vi "Tool STroker analog Variables.vi"(11 "error in (no error)":errorcluster, 12 "Tool folder name":string) -> (15 "error out":errorcluster)   [LabVIEW 2011]
uses:
  Measurments Handling/Fixed Digital Channel Definition.ctl
  Measurments Handling/Update frequensies.ctl
  Measurments Handling/Channel catagory Enum.ctl
  Variable List Stroker Digital2.ctl
  Tool/Extended channel identifier for tool.ctl
  Variable List Stroker Analog2.ctl
  Measurments Handling/Fixed Analog Channel Definition.ctl
  Measurments Handling/Units/Quantity enum.ctl
  Measurments Handling/Scaling.ctl
  <vilib>/Utility/VariantDataType/GetNumericInfo.vi
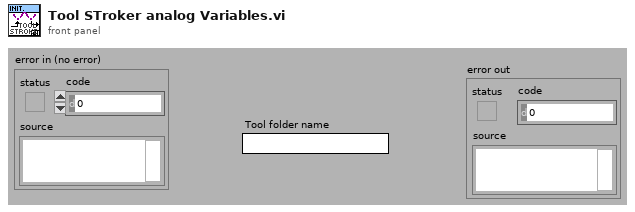
[diagram p1: front panel]
types:
  T1 = typedef "Variable List Stroker Analog2.ctl" = enum16{"Tool max Temperature", "Tool (Solenoid) Temperature", "Tool supply Voltage", "Tool (Controller) Current", "Tool Acceleration X", "Tool Acceleration Y", "Tool Acceleration Z", "Tool (Controller) Temperature", "Tool Acceleration Sum", "Tool Inclination", "Tool Rotation", "Tool Stroke Extension", "Tool GP Sensor 1", "Tool GP Sensor 2", "Tool (Pressure 1) Temperature", "Tool Pressure 1", "Tool (Pressure 2) Temperature", "Tool Pressure 2", "Do not use (SIF)", "Do not use (SOF)", "Stroke Force"}
  T2 = typedef "Fixed Analog Channel Definition.ctl" = cluster{"ID":u16, "Name":string, "Quantity":T3, "Unit":string, "Maximum upd":T4, "Comment":string, "Help file Name":string, "Help file Section ":string, "Category":T5, "User adjustable Scaling":bool, "Default Scaling":T6, "In use":bool, "Default Unit":i32}
  T3 = typedef "Quantity enum.ctl" = enum16{"Acceleration", "Angle", "Current", "Force", "Distance", "Pressure", "Resistance", "Rotational Speed", "Speed", "Temperature", "Tension", "Torque", "Voltage", "Weight"}
  T4 = typedef "Update frequensies.ctl" = enum16{"2 Hz", "1 Hz", "0.1 Hz"}
  T5 = typedef "Channel catagory Enum.ctl" = enum16{"No Category", "Power", "Temperature", "Pressure"}
  T6 = typedef "Scaling.ctl" = cluster{"Gain":dbl, "Offset":dbl}
  T7 = typedef "Extended channel identifier for tool.ctl" = cluster{"ID":T1, "Variable Defenition":T2}
  T8 = typedef "Fixed Digital Channel Definition.ctl" = cluster{"ID":u16, "Name":string, "NA Text":string, "Off Text":string, "On Text":string, "Maximum upd":T4, "Comment":string, "Help file Name":string, "Help file Section ":string, "Catagory":T5, "In use":bool}
  T9 = typedef "Variable List Stroker Digital2.ctl" = enum16{"Tool Stroke enable Valve", "Tool Stroke direction Valve", "Tool Anchor Valve", "Tool Relay 1", "Tool Relay 2", "Tool node pressure 1", "Tool node pressure 2", "Tool node solenoid", "Tool High G Monitoring", "Tool High G Recording", "Tool High G Data ready", "Tool Anchor(Not Available)", "Tool error Controller", "Tool error Pressure 1", "Tool error Pressure 2", "Tool error Solenoid", "Tool stopped Controller", "Tool stopped Pressure 1", "Tool stopped Pressure 2", "Tool stopped Solenoid", "Stroke Target seeking", "Stroke Moving Out", "Stroke Moving Inn", "Stroke valves set for Out", "Stroke valves set for In", "Stroke In (force)", "Stroke Out (force)", "Stroke Force decreasing(in)", "Stroke Force decreasing(out)", "Stroke Force change not correct", "Stroke SLIPS established P1", "Stroke SLIPS established P2", "Stroke SLIPS established"}
  T10 = typedef "User Setting DigitalChannel.ctl" = cluster{"Responses":cluster{"Technical Error (NA)":T11, "OFF / FALSE":T13, "ON / TRUE":T13}}
  T11 = typedef "Alarm Responce.ctl" = cluster{"Action":T12, "Alarm":bool}
  T12 = typedef "Action List.ctl" = u16
  T13 = typedef "Alarm Responce dig.ctl" = cluster{"Action":T12, "Alarm":bool, "Exclamation":bool}
  T14 = typedef "User Setting Analog Channel Bg.ctl" = cluster{"Scaling":T6, "Limits and responces":T15, "Allow Graph selection by user":bool, "Unit":u16}
  T15 = typedef "Alarm Setup Analog.ctl" = cluster{"Technical Error(NA)":T11, "LL":T11, "L":T11, "H":T11, "HH":T11, "Limits":T16}
  T16 = typedef "Limits.ctl" = cluster{"LL":dbl, "L":dbl, "H":dbl, "HH":dbl}
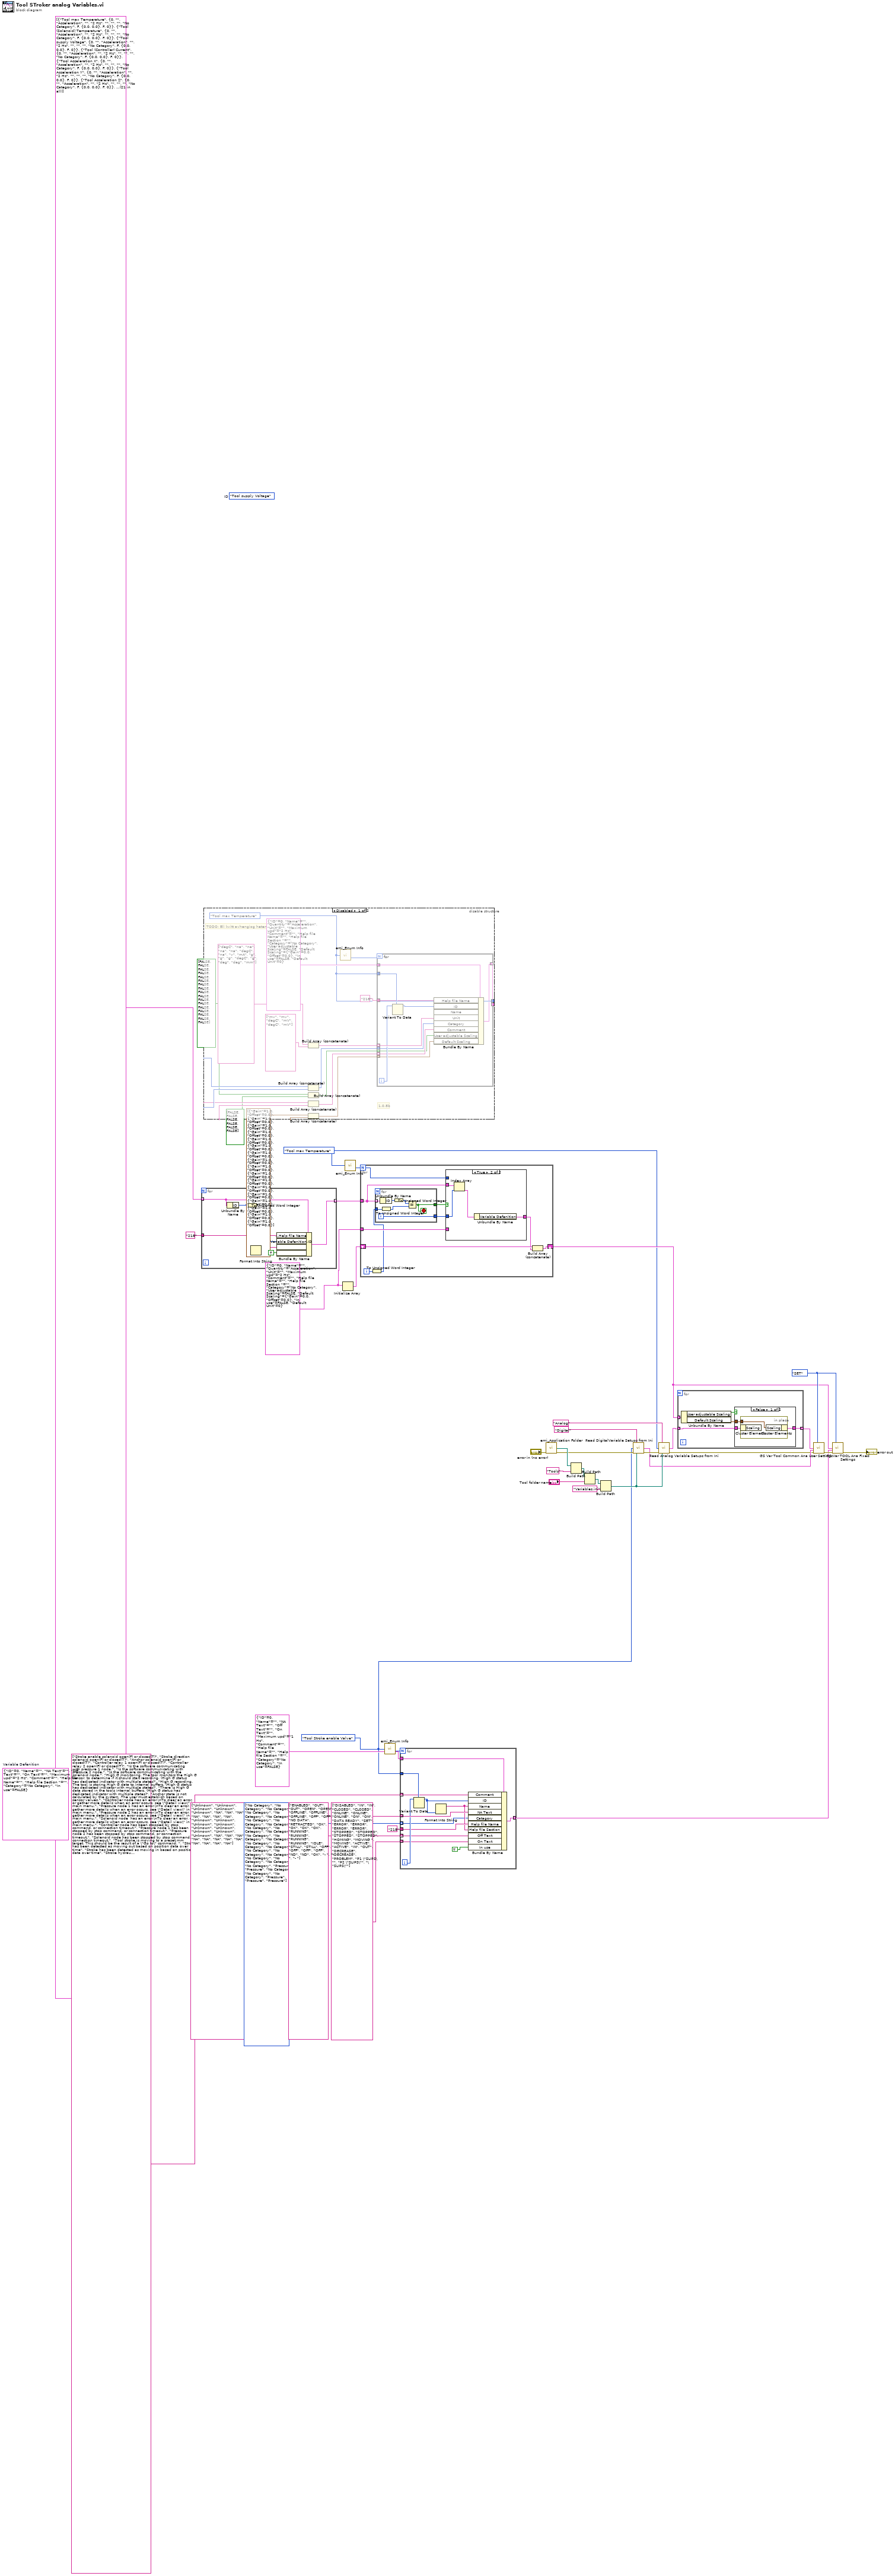
[diagram p0: block diagram]
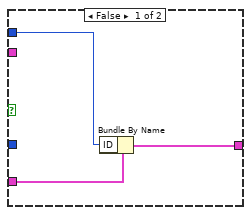
[diagram p2: hidden frame]
diagram:
  (unwired) Variable_List_Stroker_Analog2."Tool supply Voltage"  # ID
  w3 = T2 {"ID"=0, "Name"="", "Quantity"=enum."Acceleration", "Unit"="", "Maximum upd"=enum."2 Hz", "Comment"="", "Help file Name"="", "Help file Section "="", "Category"=enum."No Category", "User adjustable Scaling"=FALSE, "Default Scaling"={"Gain"=0.0, "Offset"=0.0}, "In use"=FALSE, "Default Unit"=0} ("Variable Defenition")
  w1 = Variable_List_Stroker_Analog2."Tool max Temperature" ("Action")
  (unwired) T8 {"ID"=0, "Name"="", "NA Text"="", "Off Text"="", "On Text"="", "Maximum upd"=enum."2 Hz", "Comment"="", "Help file Name"="", "Help file Section "="", "Catagory"=enum."No Category", "In use"=FALSE}  # Variable Defenition
  w22 = T5[] [enum."No Category", enum."No Category", enum."No Category", enum."No Category", enum."No Category", enum."No Category", enum."No Category", enum."No Category", enum."No Category", enum."No Category", enum."No Category", enum."No Category", enum."No Category", enum."No Category", enum."No Category", enum."No Category", enum."No Category", enum."No Category", enum."No Category", enum."No Category", enum."No Category", enum."No Category", enum."No Category", enum."No Category", enum."No Category", enum."Pressure", enum."Pressure", enum."No Category", enum."No Category", enum."No Category", enum."Pressure", enum."Pressure", enum."Pressure"] items=["No Category", "Power", "Temperature", "Pressure"]
  w14 = Variable_List_Stroker_Digital2."Tool Stroke enable Valve" ("Action")
  w29 = enum16{"GET", "SET"}."SET" ("Action(GET)")
  n1 = for {
    tunnel: T7[] [{"ID"=enum."Tool max Temperature", "Variable Defenition"={"ID"=0, "Name"="", "Quantity"=enum."Acceleration", "Unit"="", "Maximum upd"=enum."2 Hz", "Comment"="", "Help file Name"="", "Help file Section "="", "Category"=enum."No Category", "User adjustable Scaling"=FALSE, "Default Scaling"={"Gain"=0.0, "Offset"=0.0}, "In use"=FALSE, "Default Unit"=0}}, {"ID"=enum."Tool (Solenoid) Temperature", "Variable Defenition"={"ID"=0, "Name"="", "Quantity"=enum."Acceleration", "Unit"="", "Maximum upd"=enum."2 Hz", "Comment"="", "Help file Name"="", "Help file Section "="", "Category"=enum."No Category", "User adjustable Scaling"=FALSE, "Default Scaling"={"Gain"=0.0, "Offset"=0.0}, "In use"=FALSE, "Default Unit"=0}}, {"ID"=enum."Tool supply Voltage", "Variable Defenition"={"ID"=0, "Name"="", "Quantity"=enum."Acceleration", "Unit"="", "Maximum upd"=enum."2 Hz", "Comment"="", "Help file Name"="", "Help file Section "="", "Category"=enum."No Category", "User adjustable Scaling"=FALSE, "Default Scaling"={"Gain"=0.0, "Offset"=0.0}, "In use"=FALSE, "Default Unit"=0}}, {"ID"=enum."Tool (Controller) Current", "Variable Defenition"={"ID"=0, "Name"="", "Quantity"=enum."Acceleration", "Unit"="", "Maximum upd"=enum."2 Hz", "Comment"="", "Help file Name"="", "Help file Section "="", "Category"=enum."No Category", "User adjustable Scaling"=FALSE, "Default Scaling"={"Gain"=0.0, "Offset"=0.0}, "In use"=FALSE, "Default Unit"=0}}, {"ID"=enum."Tool Acceleration X", "Variable Defenition"={"ID"=0, "Name"="", "Quantity"=enum."Acceleration", "Unit"="", "Maximum upd"=enum."2 Hz", "Comment"="", "Help file Name"="", "Help file Section "="", "Category"=enum."No Category", "User adjustable Scaling"=FALSE, "Default Scaling"={"Gain"=0.0, "Offset"=0.0}, "In use"=FALSE, "Default Unit"=0}}, {"ID"=enum."Tool Acceleration Y", "Variable Defenition"={"ID"=0, "Name"="", "Quantity"=enum."Acceleration", "Unit"="", "Maximum upd"=enum."2 Hz", "Comment"="", "Help file Name"="", "Help file Section "="", "Category"=enum."No Category", "User adjustable Scaling"=FALSE, "Default Scaling"={"Gain"=0.0, "Offset"=0.0}, "In use"=FALSE, "Default Unit"=0}}, {"ID"=enum."Tool Acceleration Z", "Variable Defenition"={"ID"=0, "Name"="", "Quantity"=enum."Acceleration", "Unit"="", "Maximum upd"=enum."2 Hz", "Comment"="", "Help file Name"="", "Help file Section "="", "Category"=enum."No Category", "User adjustable Scaling"=FALSE, "Default Scaling"={"Gain"=0.0, "Offset"=0.0}, "In use"=FALSE, "Default Unit"=0}}, {"ID"=enum."Tool (Controller) Temperature", "Variable Defenition"={"ID"=0, "Name"="", "Quantity"=enum."Acceleration", "Unit"="", "Maximum upd"=enum."2 Hz", "Comment"="", "Help file Name"="", "Help file Section "="", "Category"=enum."No Category", "User adjustable Scaling"=FALSE, "Default Scaling"={"Gain"=0.0, "Offset"=0.0}, "In use"=FALSE, "Default Unit"=0}}, {"ID"=enum."Tool Acceleration Sum", "Variable Defenition"={"ID"=0, "Name"="", "Quantity"=enum."Acceleration", "Unit"="", "Maximum upd"=enum."2 Hz", "Comment"="", "Help file Name"="", "Help file Section "="", "Category"=enum."No Category", "User adjustable Scaling"=FALSE, "Default Scaling"={"Gain"=0.0, "Offset"=0.0}, "In use"=FALSE, "Default Unit"=0}}, {"ID"=enum."Tool Inclination", "Variable Defenition"={"ID"=0, "Name"="", "Quantity"=enum."Acceleration", "Unit"="", "Maximum upd"=enum."2 Hz", "Comment"="", "Help file Name"="", "Help file Section "="", "Category"=enum."No Category", "User adjustable Scaling"=FALSE, "Default Scaling"={"Gain"=0.0, "Offset"=0.0}, "In use"=FALSE, "Default Unit"=0}}, {"ID"=enum."Tool Rotation", "Variable Defenition"={"ID"=0, "Name"="", "Quantity"=enum."Acceleration", "Unit"="", "Maximum upd"=enum."2 Hz", "Comment"="", "Help file Name"="", "Help file Section "="", "Category"=enum."No Category", "User adjustable Scaling"=FALSE, "Default Scaling"={"Gain"=0.0, "Offset"=0.0}, "In use"=FALSE, "Default Unit"=0}}, {"ID"=enum."Tool Stroke Extension", "Variable Defenition"={"ID"=0, "Name"="", "Quantity"=enum."Acceleration", "Unit"="", "Maximum upd"=enum."2 Hz", "Comment"="", "Help file Name"="", "Help file Section "="", "Category"=enum."No Category", "User adjustable Scaling"=FALSE, "Default Scaling"={"Gain"=0.0, "Offset"=0.0}, "In use"=FALSE, "Default Unit"=0}}, {"ID"=enum."Tool GP Sensor 1", "Variable Defenition"={"ID"=0, "Name"="", "Quantity"=enum."Acceleration", "Unit"="", "Maximum upd"=enum."2 Hz", "Comment"="", "Help file Name"="", "Help file Section "="", "Category"=enum."No Category", "User adjustable Scaling"=FALSE, "Default Scaling"={"Gain"=0.0, "Offset"=0.0}, "In use"=FALSE, "Default Unit"=0}}, {"ID"=enum."Tool GP Sensor 2", "Variable Defenition"={"ID"=0, "Name"="", "Quantity"=enum."Acceleration", "Unit"="", "Maximum upd"=enum."2 Hz", "Comment"="", "Help file Name"="", "Help file Section "="", "Category"=enum."No Category", "User adjustable Scaling"=FALSE, "Default Scaling"={"Gain"=0.0, "Offset"=0.0}, "In use"=FALSE, "Default Unit"=0}}, {"ID"=enum."Tool (Pressure 1) Temperature", "Variable Defenition"={"ID"=0, "Name"="", "Quantity"=enum."Acceleration", "Unit"="", "Maximum upd"=enum."2 Hz", "Comment"="", "Help file Name"="", "Help file Section "="", "Category"=enum."No Category", "User adjustable Scaling"=FALSE, "Default Scaling"={"Gain"=0.0, "Offset"=0.0}, "In use"=FALSE, "Default Unit"=0}}, {"ID"=enum."Tool Pressure 1", "Variable Defenition"={"ID"=0, "Name"="", "Quantity"=enum."Acceleration", "Unit"="", "Maximum upd"=enum."2 Hz", "Comment"="", "Help file Name"="", "Help file Section "="", "Category"=enum."No Category", "User adjustable Scaling"=FALSE, "Default Scaling"={"Gain"=0.0, "Offset"=0.0}, "In use"=FALSE, "Default Unit"=0}}, {"ID"=enum."Tool (Pressure 2) Temperature", "Variable Defenition"={"ID"=0, "Name"="", "Quantity"=enum."Acceleration", "Unit"="", "Maximum upd"=enum."2 Hz", "Comment"="", "Help file Name"="", "Help file Section "="", "Category"=enum."No Category", "User adjustable Scaling"=FALSE, "Default Scaling"={"Gain"=0.0, "Offset"=0.0}, "In use"=FALSE, "Default Unit"=0}}, {"ID"=enum."Tool Pressure 2", "Variable Defenition"={"ID"=0, "Name"="", "Quantity"=enum."Acceleration", "Unit"="", "Maximum upd"=enum."2 Hz", "Comment"="", "Help file Name"="", "Help file Section "="", "Category"=enum."No Category", "User adjustable Scaling"=FALSE, "Default Scaling"={"Gain"=0.0, "Offset"=0.0}, "In use"=FALSE, "Default Unit"=0}}, {"ID"=enum."Do not use (SIF)", "Variable Defenition"={"ID"=0, "Name"="", "Quantity"=enum."Acceleration", "Unit"="", "Maximum upd"=enum."2 Hz", "Comment"="", "Help file Name"="", "Help file Section "="", "Category"=enum."No Category", "User adjustable Scaling"=FALSE, "Default Scaling"={"Gain"=0.0, "Offset"=0.0}, "In use"=FALSE, "Default Unit"=0}}, {"ID"=enum."Do not use (SOF)", "Variable Defenition"={"ID"=0, "Name"="", "Quantity"=enum."Acceleration", "Unit"="", "Maximum upd"=enum."2 Hz", "Comment"="", "Help file Name"="", "Help file Section "="", "Category"=enum."No Category", "User adjustable Scaling"=FALSE, "Default Scaling"={"Gain"=0.0, "Offset"=0.0}, "In use"=FALSE, "Default Unit"=0}}, {"ID"=enum."Stroke Force", "Variable Defenition"={"ID"=0, "Name"="", "Quantity"=enum."Acceleration", "Unit"="", "Maximum upd"=enum."2 Hz", "Comment"="", "Help file Name"="", "Help file Section "="", "Category"=enum."No Category", "User adjustable Scaling"=FALSE, "Default Scaling"={"Gain"=0.0, "Offset"=0.0}, "In use"=FALSE, "Default Unit"=0}}] -> [w43] mode=indexing
    tunnel: "218" ("Help file Name") -> [w44]
    tunnel: [w38] -> w5 mode=indexing
    n2 = Unbundle By Name(w43) -> ("ID"=w41:T1)
    n3 = To Unsigned Word Integer(number=w41) -> (unsigned 16bit integer=w42:u16)
    n4 = Format Into String(w41) -> (resulting string=w40:string)  [unwired: 3 in, 1 out]
    n5 = Bundle By Name(cluster=w43, "Variable Defenition.Help file Name"=w44, "Variable Defenition.ID"=w42, "Variable Defenition.Name"=w40, "Variable Defenition.In use"=TRUE) -> (w38:T7)
  }
  n6 = disable-structure shown="Disabled" {
    disable-tunnel: [w46 _] -> _
    disable-tunnel: [w45 _] -> _
    frame Disabled {
      w58 = T5[] [enum."No Category", enum."No Category", enum."Temperature", enum."Pressure", enum."Temperature", enum."Pressure"] items=["No Category", "Power", "Temperature", "Pressure"]
      w59 = T5[] [enum."Temperature", enum."No Category", enum."No Category", enum."No Category", enum."No Category", enum."Temperature", enum."No Category", enum."Power", enum."Power", enum."No Category", enum."No Category", enum."No Category", enum."Temperature", enum."No Category", enum."No Category", enum."No Category", enum."No Category"] items=["No Category", "Power", "Temperature", "Pressure"]
      w45 = Variable_List_Stroker_Analog2."Tool max Temperature" ("Action")
      # "1.0.8b"
      # "TODO: Bli kvitt avhengiog heten av denne"
      n7 = Build Array (concatenate)(string[] ["degC", "na", "na", "na", "na", "degC", "na", "v", "mA", "g", "g", "g", "degC", "g", "deg", "deg", "mm"], string[] ["mv", "mv", "degC", "mV", "degC", "mV"]) -> (w61:string[])
      n8 = Build Array (concatenate)(w59, w58) -> (w54:T5[])
      n9 = Build Array (concatenate)(bool[] [FALSE, FALSE, FALSE, FALSE, FALSE, FALSE, FALSE, FALSE, FALSE, FALSE, FALSE, FALSE, FALSE, FALSE, FALSE, FALSE, FALSE], bool[] [FALSE, FALSE, FALSE, FALSE, FALSE, FALSE]) -> (w51:bool[])
      n10 = Build Array (concatenate)(string[] ["The Highest temperature currently beeing measured in the tool.\nIf data from any of the tools temperature sensors is not reporting data, this is reported as Not Available.", "Not available\n", "Not available\n", "Not available\n", "Not available\n", "Temperature of the Solonoid electronics", "Not availabe\nThe Downhole Power Supply Temperature", "The Downhole tool's Controller board input voltage", "The Downhole tool's controller board input current", "The Downhole tool's controller board Acceleromter X axis. Used to determin heading", "The Downhole tool's controller board Acceleromter Y axis. Used to determin heading", "The Downhole tool's controller board Acceleromter Z axis. Used to determin heading", "The Downhole tool's controller board temperature", "Sum of the accelerations detected by the Downhole tool processor board", "Tool inclination as calculated by the controller board's accelerometer", "Tool rotation as calculated by the controller board's accelerometer", "Not available\nTool rotational speed  as calculated by the controller board's accelerometer"], string[] ["Tool Controller AI 24bit bridge sensor 1", "Tool Controller AI 24bit bridge sensor 2", "Pressure node 1 temperature", "Pressure node 1, pressure (shown in mV input of the sensor)", "Pressure node 2 temperature", "Pressure node 2, pressure (shown in mV input of the sensor)"]) -> (w55:string[])
      n11 = Build Array (concatenate)(T6[] [{"Gain"=1.0, "Offset"=0.0}, {"Gain"=1.0, "Offset"=0.0}, {"Gain"=1.0, "Offset"=0.0}, {"Gain"=1.0, "Offset"=0.0}, {"Gain"=1.0, "Offset"=0.0}, {"Gain"=1.0, "Offset"=0.0}, {"Gain"=1.0, "Offset"=0.0}, {"Gain"=1.0, "Offset"=0.0}, {"Gain"=1.0, "Offset"=0.0}, {"Gain"=1.0, "Offset"=0.0}, {"Gain"=1.0, "Offset"=0.0}, {"Gain"=1.0, "Offset"=0.0}, {"Gain"=1.0, "Offset"=0.0}, {"Gain"=1.0, "Offset"=0.0}, {"Gain"=1.0, "Offset"=0.0}, {"Gain"=1.0, "Offset"=0.0}, {"Gain"=1.0, "Offset"=0.0}], T6[] [{"Gain"=1.0, "Offset"=0.0}, {"Gain"=1.0, "Offset"=0.0}, {"Gain"=1.0, "Offset"=0.0}, {"Gain"=1.0, "Offset"=0.0}, {"Gain"=1.0, "Offset"=0.0}, {"Gain"=1.0, "Offset"=0.0}]) -> (w48:T6[])
      n12 = call "emi_Enum Info.vi"("Enum"=w45) -> ("Numb Elements"=w62:i32)  [unwired: 11 in, 3 out]
      n13 = for {
        N: w62 -> [_]
        tunnel: w45 -> [w76]
        tunnel: T2 {"ID"=0, "Name"="", "Quantity"=enum."Acceleration", "Unit"="", "Maximum upd"=enum."2 Hz", "Comment"="", "Help file Name"="", "Help file Section "="", "Category"=enum."No Category", "User adjustable Scaling"=FALSE, "Default Scaling"={"Gain"=0.0, "Offset"=0.0}, "In use"=FALSE, "Default Unit"=0} ("Variable Defenition") -> [w72]
        tunnel: [w73] -> w46 mode=indexing
        tunnel: w61 -> [w71] mode=indexing
        tunnel: w54 -> [w69] mode=indexing
        tunnel: w55 -> [w68] mode=indexing
        tunnel: w51 -> [w67] mode=indexing
        tunnel: w48 -> [w66] mode=indexing
        tunnel: "218" ("Help file Name") -> [w65]
        i -> [w70]
        n14 = Variant To Data(type=w76, Variant=w70) -> (data=w74:T1)  [unwired: 1 in, 1 out]
        n15 = Bundle By Name(cluster=w72, "Help file Name"=w65, "ID"=w74, "Unit"=w71, "Category"=w69, "Comment"=w68, "User adjustable Scaling"=w67, "Default Scaling"=w66) -> (w73:T2, "Name"=w75:string)
      }
    }
    frame Enabled {
    }
  }
  n16 = Initialize Array(w3) -> (w4:T2[])  [unwired: 1 in]
  n17 = call "emi_Enum Info.vi"("Enum"=w1) -> ("Numb Elements"=w6:i32)  [unwired: 11 in, 3 out]
  n18 = for {
    N: w6 -> [w78]
    tunnel: w5 -> [w85]
    shift-right: [w81] -> w2
    shift-left: w4 -> [w82]
    tunnel: w3 -> [w80]
    i -> [w86]
    n19 = To Unsigned Word Integer(number=w86) -> (unsigned 16bit integer=w77:u16)
    n20 = for {
      tunnel: w85 -> [w100] mode=indexing
      tunnel: w77 -> [w97]
      tunnel: [w95] -> w83
      tunnel: [w94] -> w84
      i -> [w94]
      stop <- w95 stop-if-true
      n21 = Unbundle By Name(w100) -> ("ID"=w98:T1)
      n22 = To Unsigned Word Integer(number=w97) -> (unsigned 16bit integer=w96:u16)
      n23 = To Unsigned Word Integer(number=w98) -> (unsigned 16bit integer=w99:u16)
      n24 = Equal?(x=w99, y=w96) -> (x = y?=w95:bool)
    }
    n25 = case shown="True" w83 {
      tunnel: w85 -> [_ w93]
      tunnel: w84 -> [_ w92]
      tunnel: w80 -> [w89 _]
      tunnel: w78 -> [w88 _]
      tunnel: [w87 w90] -> w79
      frame False {
        n26 = Bundle By Name(cluster=w89, "ID"=w88) -> (w87:T2)
      }
      frame True {
        n27 = Index Array(array=w93, index=w92) -> (element=w91:T7)
        n28 = Unbundle By Name(w91) -> ("Variable Defenition"=w90:T2)
      }
    }
    n29 = Build Array (concatenate)(w82, w79) -> (w81:T2[])
  }
  n30 = call "emi_Enum Info.vi"("Enum"=w14) -> ("Numb Elements"=w25:i32)  [unwired: 11 in, 3 out]
  n31 = for {
    N: w25 -> [_]
    tunnel: w14 -> [w113]
    tunnel: T8 {"ID"=0, "Name"="", "NA Text"="", "Off Text"="", "On Text"="", "Maximum upd"=enum."1 Hz", "Comment"="", "Help file Name"="", "Help file Section "="", "Catagory"=enum."No Category", "In use"=FALSE} ("Variable Defenition") -> [w110]
    tunnel: [w111] -> w12 mode=indexing
    tunnel: string[] ["Unknown", "Unknown", "Unknown", "Unknown", "Unknown", "NA", "NA", "NA", "NA", "NA", "NA", "NA", "Unknown", "Unknown", "Unknown", "Unknown", "Unknown", "Unknown", "Unknown", "Unknown", "Unknown", "NA", "NA", "NA", "NA", "NA", "NA", "NA", "NA", "NA", "NA", "NA", "NA"] -> [w109] mode=indexing
    tunnel: w22 -> [w105] mode=indexing
    tunnel: "218" -> [w107]
    tunnel: string[] ["ENABLED", "OUT", "OUT", "OPEN", "OPEN", "OFFLINE", "OFFLINE", "OFFLINE", "OFF", "OFF", "NO DATA", "RETRACTED", "OK", "OK", "OK", "OK", "RUNNING", "RUNNING", "RUNNING", "RUNNING", "IDLE", "STILL", "STILL", "OFF", "OFF", "OFF", "OFF", "ND", "ND", "OK", "- ", "- ", "- "] -> [w104] mode=indexing
    tunnel: string[] ["DISABLED", "IN", "IN", "CLOSED", "CLOSED", "ONLINE", "ONLINE", "ONLINE", "ON", "ON", "DATA READY", "SET", "ERROR", "ERROR", "ERROR", "ERROR", "STOPPED", "STOPPED", "STOPPED", "STOPPED", "HOMING", "MOVING ", "MOVING", "ACTIVE", "ACTIVE", "IN", "OUT", "DECREASE", "DECREASE", "PROBLEM", "P1 \"SLIPS\"", "P2 \"SLIPS\"", "\"SLIPS\""] -> [w103] mode=indexing
    tunnel: string[] ["Stroke enable solenoid open(F) or closed(T)", "Stroke direction solenoid open(F) or closed(T)", "Anchor solenoid open(F) or closed(T)", "Controller relay 1 open(F) or closed(T)", "Controller relay 2 open(F) or closed(T)", "Is the software communicating with pressure 1 node.", "Is the software communicating with pressure 2 node.", "Is the software communicating with the solenoid node.", "High G monitoring. The tool monitors the High G sensor, to determine if it should start recording. (High G status has dedicated indicator with multiple states)", "High G recording. The tool is storing High G data to internal buffers. (High G status has dedicated indicator with multiple states)", "There is High G data stored in the tools internal buffers. (High G status has dedicated indicator with multiple states)", "Anchor state is not calculated by the system .The user must establish based on sensor values.", "Controller node has an error.\nTo clear an error, or gather more details when an error occurs, see \"Detail view\" in main menu.", "Pressure node 1 has an error.\nTo clear an error, or gather more details when an error occurs, see \"Detail view\" in main menu.", "Pressure node 2 has an error.\nTo clear an error, or gather more details when an error occurs, see \"Detail view\" in main menu.", "Solenoid node  has an error.\nTo clear an error, or gather more details when an error occurs, see \"Detail view\" in main menu.", "Controller node has been stopped by stop command, or connection timeout.", "Pressure node 1 has been stopped by stop command, or connection timeout.", "Pressure node 2 has been stopped by stop command, or connection timeout.", "Solenoid node has been stopped by stop command, or connection timeout.", "Tool stroke is moving to a preset mm target. This should be the result of a \"Go to\" command. ", "Stroke has been detected as moving out based on position data over time", "Stroke has been detected as moving in based on position data over time", "Stroke hydraulic valves are positioned to move the stroke out.", "Stroke hydraulic valves are positioned to move the stroke in.", "Pressure readings are indicating that the stroke is moving in", "Pressure readings are indicating that the stroke is moving out", "Pressure readings are indicating that the inward stroke force is decreasing. ", "Pressure readings are indicating that the outward stroke force is decreasing. ", "Stroke force is decreasing when it should be increasing. \nExpected: When pressure is over limit to indicate movement, and valves are set for movement, the pressure on the stroking side is not expected to fall.", "Pressure node 1 indicates that SLIPS has been established.", "Pressure node 2 indicates that SLIPS has been established.", "Both pressure nodes indicate that SLIPS has been established."] -> [w102] mode=indexing
    i -> [w108]
    n32 = Variant To Data(type=w113, Variant=w108) -> (data=w112:T9)  [unwired: 1 in, 1 out]
    n33 = Format Into String(w112) -> (resulting string=w106:string)  [unwired: 3 in, 1 out]
    n34 = Bundle By Name(cluster=w110, "Comment"=w102, "ID"=w112, "Name"=w106, "NA Text"=w109, "Catagory"=w105, "Help file Name"=w107, "Help file Section"=w106, "Off Text"=w104, "On Text"=w103, "In use"=TRUE) -> (w111:T8)
  }
  n35 = call "emi_Application Folder.vi"("error in (no error)"="error in (no error)") -> ("Dir"=w27:path, "error out"=w18:errorcluster)  [unwired: 13 in]
  n36 = Build Path(base path=w27, name or relative path="Tools") -> (appended path=w32:path)
  n37 = Build Path(base path=w32, name or relative path="Tool folder name") -> (appended path=w34:path)
  n38 = Build Path(base path=w34, name or relative path="Variables.ini") -> (appended path=w16:path)
  n39 = call "Read DigitalVariable Setups from Ini.vi"("error in (no error)"=w18, "Path"=w16, "Enum with Variable List"=w14, "Section(\"Default\")"="Digital" ("Section(\"Default\")")) -> ("error out"=w17:errorcluster, "Digitale User settigns"=w13:T10[])  [unwired: 10 in]
  n40 = call "Read Analog Variable Setups from Ini.vi"("error in (no error)"=w17, "Path"=w16, "Enum with Variable List"=w1, "Section(\"Default\")"="Analog" ("Section(\"Default\")")) -> ("error out"=w11:errorcluster, "Analog User settigns"=w10:T14[])  [unwired: 9 in, 1 out]
  n41 = for {
    tunnel: w10 -> [w118] mode=indexing
    tunnel: [w114] -> w9 mode=indexing
    tunnel: w2 -> [w117] mode=indexing
    n42 = Unbundle By Name(w117) -> ("User adjustable Scaling"=w115:bool, "Default Scaling"=w116:T6)
    n43 = case shown="False" w115 {
      tunnel: w118 -> [w121 w123]
      tunnel: w116 -> [w120 _]
      tunnel: [w119 w123] -> w114
      frame False {
        n44 = in-place {
          in-place-border: w120 -> [w122]
          n45 = in-place-cluster #1(w121) -> ()  [unwired: 1 out]
          n46 = in-place-cluster #1("Scaling"=w122) -> (w119:T14)
        }
      }
      frame True {
      }
    }
  }
  n47 = call "GS Var Tool Common Ana User Settings.vi"("Action(GET)"=w29, "Tool analog var User settigns in"=w9, "Tool digital var User settigns in"=w13, "error in (no error)"=w11) -> ("error out"=w31:errorcluster)  [unwired: 9 in, 2 out]
  n48 = call "GS Var TOOL Ana Fixed Settings.vi"("Action(GET)"=w29, "Tool Analog Var Fixed in"=w2, "Tool Digital Var Fixed in"=w12, "error in (no error)"=w31) -> ("error out"=→"error out":errorcluster)  [unwired: 9 in, 2 out]
